vi "Status Logger FGV.vi"(7 "Action":T1=enum."Get file path", 8 "error in (no error)":errorcluster, 10 "Status":string) -> (0 "error out":errorcluster, 3 "Staus Log Path":path)   [LabVIEW 2015]
uses:
  Status Log.ctl
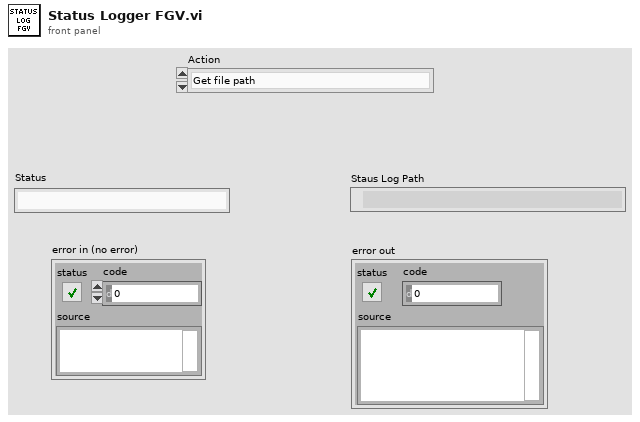
[diagram p1: front panel]
types:
  T1 = typedef "Status Log.ctl" = enum16{"Close file", "Open Status file", "Add Status", "Get file path"}
  T2 = enum16{"open", "replace", "create", "open or create", "replace or create", "replace or create with confirmation"}
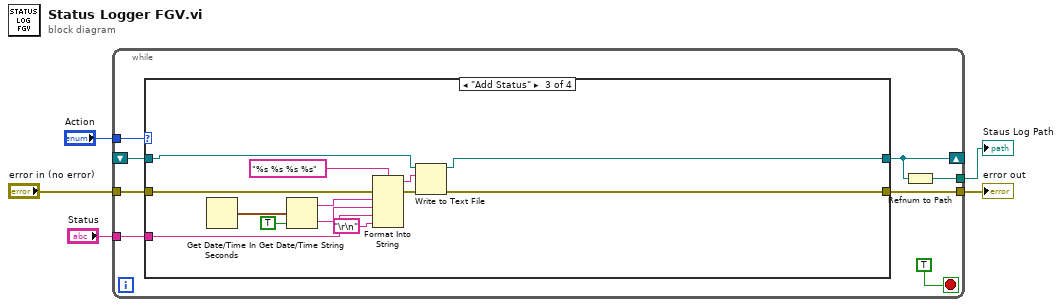
[diagram p0: block diagram]
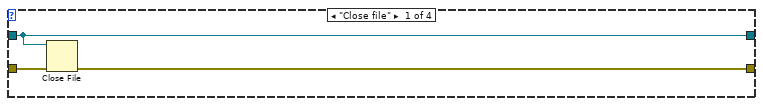
[diagram p2: hidden frame]
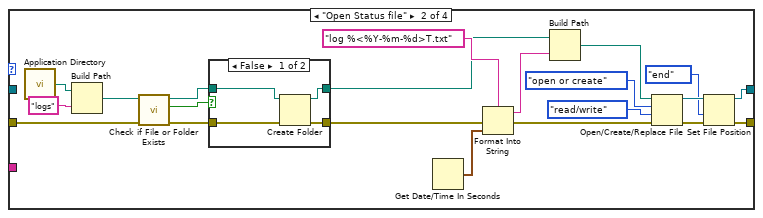
[diagram p3: hidden frame]
diagram:
  n1 = while {
    tunnel: "Action" -> [w12]
    tunnel: "Status" -> [w11]
    tunnel: [w10] -> w3
    tunnel: "error in (no error)" -> [w9]
    shift-right: [w6] -> _
    shift-left: _ -> [w8]
    tunnel: [w7] -> w1
    stop <- TRUE stop-if-true
    n2 = case shown="\"Add Status\"" w12 {
      tunnel: w11 -> [_ _ w50 _]
      tunnel: [w15 w26 w47 w58] -> w10
      tunnel: w9 -> [w16 w18 w56 w58]
      tunnel: [w14 w25 w44 w57] -> w6
      tunnel: w8 -> [w14 _ w46 w57]
      frame "Close file" {
        n3 = Close File(refnum=w14, error in=w16) -> (error out=w15:errorcluster)  [unwired: 1 out]
      }
      frame "Open Status file" {
        n4 = call <vilib>:"Application Directory.vi"() -> ("Application Directory"=w37:path)
        n5 = Build Path(base path=w37, name or relative path="logs") -> (appended path=w23:path)
        n6 = call <vilib>:"Check if File or Folder Exists.vi"("error in (no error)"=w18, "path"=w23) -> ("error out"=w19:errorcluster, "file or folder exists?"=w22:bool, "dup path"=w21:path)  [unwired: 7 in]
        n7 = case shown="False" w22 {
          tunnel: w21 -> [w41 w43]
          tunnel: [w40 w43] -> w20
          tunnel: w19 -> [w39 w42]
          tunnel: [w38 w42] -> w17
          frame False {
            n8 = Create Folder(path (use dialog)=w41, error in=w39) -> (created path=w40:path, error out=w38:errorcluster)  [unwired: 1 in, 1 out]
          }
          frame True {
          }
        }
        n9 = Get Date/Time In Seconds() -> (seconds since 1Jan1904=w35:timestamp)
        n10 = Format Into String(format string="log %<%Y-%m-%d>T.txt", error in=w17, w35) -> (resulting string=w33:string, error out=w34:errorcluster)  [unwired: 1 in]
        n11 = Build Path(base path=w20, name or relative path=w33) -> (appended path=w32:path)
        n12 = Open/Create/Replace File(file path (use dialog)=w32, error in=w34, operation (0:open)=T2."open or create", access (0:read/write)=enum16{"read/write", "read-only", "write-only"}."read/write") -> (refnum out=w27:refnum<file>, error out=w28:errorcluster)  [unwired: 2 in, 1 out]
        n13 = Set File Position(refnum=w27, from (0:start)=enum16{"start", "end", "current"}."end", error in=w28) -> (refnum out=w25:refnum<file>, error out=w26:errorcluster)  [unwired: 1 in]
      }
      frame "Add Status" {
        n14 = Get Date/Time In Seconds() -> (seconds since 1Jan1904=w54:timestamp)
        n15 = Get Date/Time String(seconds (now)=w54, want seconds? (F)=TRUE) -> (date string=w52:string, time string=w51:string)  [unwired: 1 in]
        n16 = Format Into String(format string="%s %s %s %s", error in=w56, w52, w51, w50, "\r\n") -> (resulting string=w45:string, error out=w48:errorcluster)  [unwired: 1 in]
        n17 = Write to Text File(file (use dialog)=w46, text=w45, error in=w48) -> (refnum out=w44:refnum<file>, error out=w47:errorcluster)  [unwired: 1 in, 1 out]
      }
      frame "Get file path" {
      }
    }
    n18 = Refnum to Path(1:w6) -> (0:w7:path)
  }
  "error out" <- w3
  "Staus Log Path" <- w1
